vi "Extended User Data.vi"(7 "Action":u16(ring) items=["Read", "Write"], 8 "Error In (no error)":errorcluster, 10 "Default Group Name In":string, 11 "VISA resource name in":refnum<visa-resource-name>) -> (0 "Error Out":errorcluster, 2 "Default Group Name Out":string, 3 "VISA resource name out":refnum<visa-resource-name>)   [LabVIEW 2020, in "Agilent 90000 Series.lvlib"]
doc: "Writes, reads, and clears data of the type User Data In to the connected VISA session."
uses:
  Agilent 90000 Series.lvlib
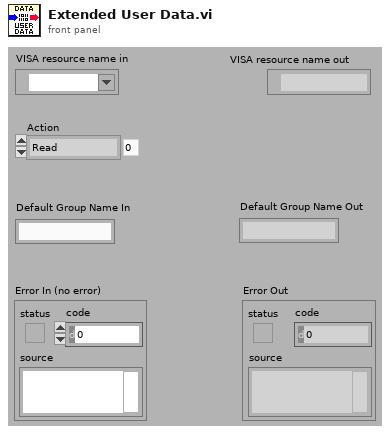
[diagram p1: front panel]
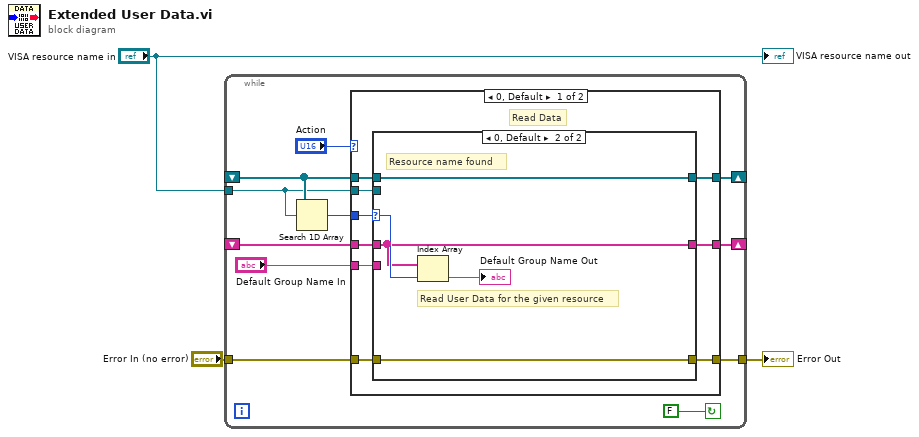
[diagram p0: block diagram]
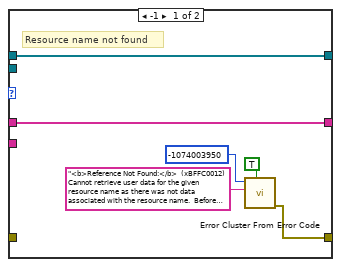
[diagram p2: hidden frame]
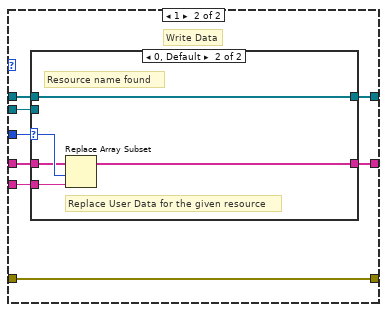
[diagram p3: hidden frame]
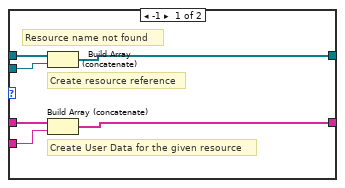
[diagram p4: hidden frame]
diagram:
  n1 = while {
    shift-right: [w11] -> _
    shift-left: _ -> [w12]
    shift-right: [w4] -> _
    shift-left: _ -> [w14]
    tunnel: "VISA resource name in" -> [w10]
    tunnel: "Error In (no error)" -> [w7]
    tunnel: [w6] -> w1
    stop <- FALSE continue-if-true
    n2 = Search 1D Array(1D array=w12, element=w10) -> (index of element=w13:i32)  [unwired: 1 in]
    n3 = case shown="0, Default" "Action" {
      tunnel: "Default Group Name In" -> [w23 w42]
      tunnel: w14 -> [w22 w41]
      tunnel: [w15 w40] -> w4
      tunnel: w13 -> [w21 w39]
      tunnel: w12 -> [w20 w38]
      tunnel: [w19 w37] -> w11
      tunnel: w10 -> [w18 w36]
      tunnel: w7 -> [w16 w35]
      tunnel: [w17 w35] -> w6
      frame 0, Default {
        # "Read Data"
        n4 = case shown="0, Default" w21 {
          selector: w21 -> [_ w34]
          tunnel: w23 -> [_ _]
          tunnel: [w28 w30] -> w15
          tunnel: w22 -> [w28 w30]
          tunnel: w20 -> [w29 w33]
          tunnel: [w29 w33] -> w19
          tunnel: w18 -> [_ _]
          tunnel: [w27 w32] -> w17
          tunnel: w16 -> [_ w32]
          frame -1 {
            # "Resource name not found"
            n5 = call <vilib>:"Error Cluster From Error Code.vi"("show call chain? (False)"=TRUE, "error message (\"\")"="<b>Reference Not Found:</b>  (xBFFC0012) Cannot retrieve user data for the given resource name as there was not data associated with the resource name.  Before you can read data, you need to write the user data using the Write Data action of this User Data VI. ", "error code (0)"=-1074003950 ("Code")) -> ("error out"=w27:errorcluster)  [unwired: 6 in]
          }
          frame 0, Default {
            # "Read User Data for the given resource"
            # "Resource name found"
            n6 = Index Array(array=w30, index=w34) -> (element=→"Default Group Name Out":string)
          }
        }
      }
      frame 1 {
        # "Write Data"
        n7 = case shown="0, Default" w39 {
          selector: w39 -> [_ w51]
          tunnel: w42 -> [w46 w52]
          tunnel: [w45 w53] -> w40
          tunnel: w41 -> [w47 w49]
          tunnel: w38 -> [w48 w50]
          tunnel: [w43 w50] -> w37
          tunnel: w36 -> [w44 _]
          frame -1 {
            # "Create resource reference"
            # "Create User Data for the given resource"
            # "Resource name not found"
            n8 = Build Array (concatenate)(w48, w44) -> (w43:refnum<visa-resource-name>[])
            n9 = Build Array (concatenate)(w47, w46) -> (w45:string[])
          }
          frame 0, Default {
            # "Replace User Data for the given resource"
            # "Resource name found"
            n10 = Replace Array Subset(array=w49, new element=w52, index=w51) -> (w53:string[])
          }
        }
      }
    }
  }
  "Error Out" <- w1
  "VISA resource name out" <- "VISA resource name in"
